vi "Flatten Version JSON.vi"(8 "error in (no error)":errorcluster, 11 "version":T1) -> (0 "error out":errorcluster, 3 "version json":string)   [LabVIEW 2017, in "DSF Core.lvlib" / "Configuration Session.lvclass"]
uses:
  Configuration Session.lvclass
  Typedefs/DSF Version Info.ctl
  DSF Core.lvlib
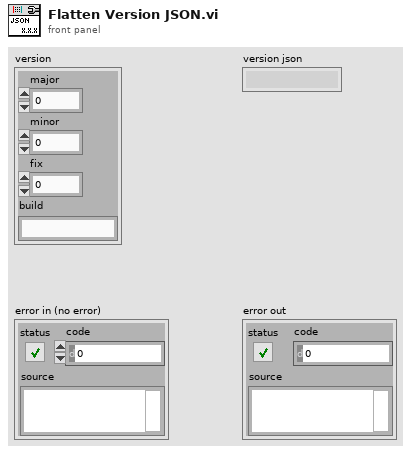
[diagram p1: front panel]
types:
  T1 = typedef "DSF Core.lvlib/DSF Version Info.ctl" = cluster{"major":u32, "minor":u32, "fix":u32, "build":string}
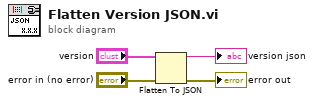
[diagram p0: block diagram]
diagram:
  n1 = Flatten To JSON(anything="version", error in (no error)="error in (no error)") -> (JSON string=→"version json":string, 11:→"error out":errorcluster)  [unwired: 1 in]
